vi "1726 Drive With PID.vi"(0 "RobotDriveDevRef in":T2, 1 "Tuning Parametres":T1 {"Acceleration Distance" min=0.0; "Minimum Speed" min=0.0 max=1.0; "Max Speed" min=0.0 max=1.0}, 2 "Target Distance":dbl, 3 "Timeout (ms)":u32) -> (7 "RobotDriveDevRef out":T2, 9 "Is Finished?":bool, 10 "Is Timedout?":bool)   [LabVIEW 2017]
uses:
  <vilib>/Rock Robotics/WPI/RobotDrive/WPI_RobotDriveDevRef.ctl
  <vilib>/Rock Robotics/WPI/MotorControl/WPI_MotorControlDeviceRef.ctl
  <vilib>/Rock Robotics/WPI/MotorControl/WPI_MotorControlType.ctl
  <vilib>/Rock Robotics/SystemInterfaces/DIO/FPGA_DIOPWMChannel.ctl
  <vilib>/Rock Robotics/WPI/PWM/WPI_PWMDeadband.ctl
  <vilib>/Rock Robotics/SystemInterfaces/DIO/FPGA_DIOChannel.ctl
  Team Code/Robot Global Data.vi
  <vilib>/addons/control/pid/pid.llb/PID (DBL).vi
  <vilib>/Rock Robotics/WPI/RobotDrive/WPI_RobotDriveArcadeDrive_Standard(NoSaturation).vi
  <vilib>/addons/control/pid/NI_PID_pid.lvlib
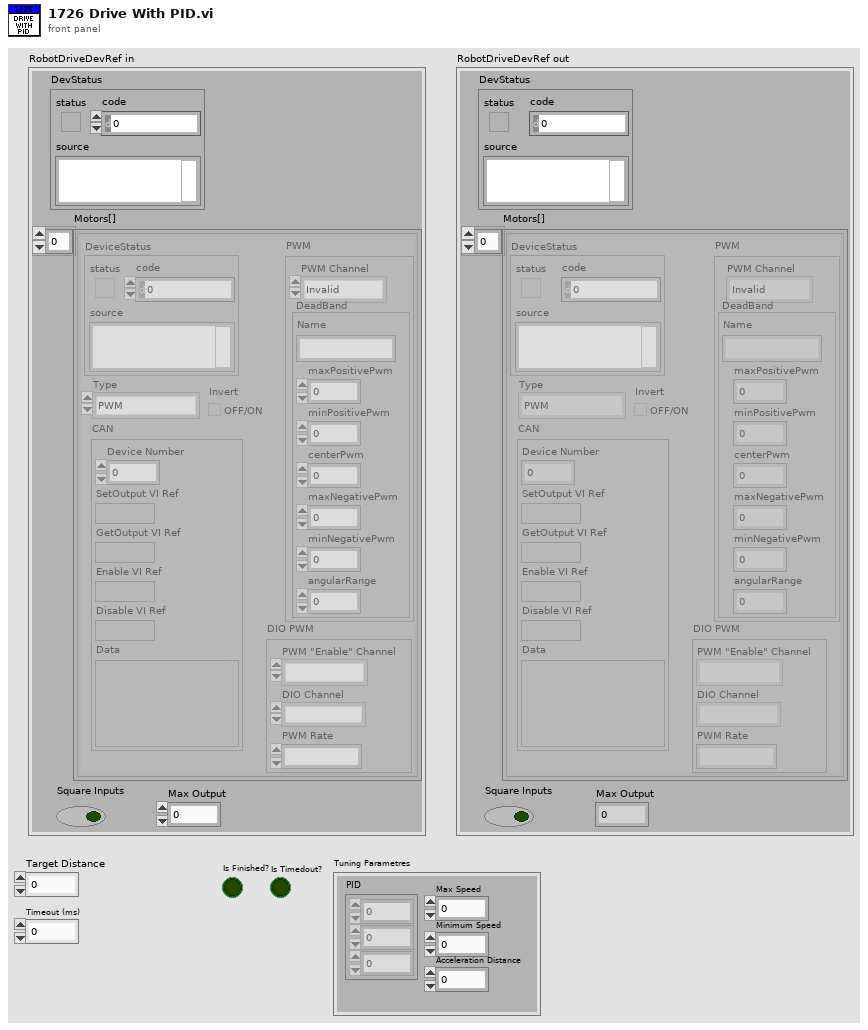
[diagram p1: front panel]
types:
  T1 = cluster{"PID":dbl[], "Max Speed":dbl, "Minimum Speed":dbl, "Acceleration Distance":dbl}
  T2 = typedef "WPI_RobotDriveDevRef.ctl" = cluster{"DevStatus":errorcluster, "Motors[]":T3[], "Square Inputs":bool, "Max Output":dbl}
  T3 = typedef "WPI_MotorControlDeviceRef.ctl" = cluster{"DeviceStatus":errorcluster, "Type":T4, "PWM":cluster{"PWM Channel":T5, "DeadBand":T6}, "CAN":cluster{"Device Number":u8, "SetOutput VI Ref":variant, "GetOutput VI Ref":variant, "Enable VI Ref":variant, "Disable VI Ref":variant, "Data":variant}, "Invert":bool, "DIO PWM":cluster{"PWM \"Enable\" Channel":T5, "DIOChannel":T7, "PWM Rate":dbl}}
  T4 = typedef "WPI_MotorControlType.ctl" = enum16{"PWM", "CAN", "DIO PWM"}
  T5 = typedef "FPGA_DIOPWMChannel.ctl" = enum8{"PWM 0", "PWM 1", "PWM 2", "PWM 3", "PWM 4", "PWM 5", "PWM 6", "PWM 7", "PWM 8", "PWM 9", "PWM MXP 0", "PWM MXP 1", "PWM MXP 2", "PWM MXP 3", "PWM MXP 4", "PWM MXP 5", "PWM MXP 6", "PWM MXP 7", "PWM MXP 8", "PWM MXP 9", "Invalid"}
  T6 = typedef "WPI_PWMDeadband.ctl" = cluster{"Name":string, "maxPositivePwm":i32, "minPositivePwm":i32, "centerPwm":i32, "maxNegativePwm":i32, "minNegativePwm":i32, "angularRange":u16}
  T7 = typedef "FPGA_DIOChannel.ctl" = enum8{"DIO 0", "DIO 1", "DIO 2", "DIO 3", "DIO 4", "DIO 5", "DIO 6", "DIO 7", "DIO 8", "DIO 9", "DIO MXP 0", "DIO MXP 1", "DIO MXP 2", "DIO MXP 3", "DIO MXP 4", "DIO MXP 5", "DIO MXP 6", "DIO MXP 7", "DIO MXP 8", "DIO MXP 9", "DIO MXP 10", "DIO MXP 11", "DIO MXP 12", "DIO MXP 13", "DIO MXP 14", "DIO MXP 15", "SPI Port CS1", "SPI Port CS2", "SPI Port CS3", "SPI Port MISO", "SPI Port MOSI", "Invalid"}
  T8 = cluster{"PID[0]":dbl, "PID[1]":dbl, "PID[2]":dbl}
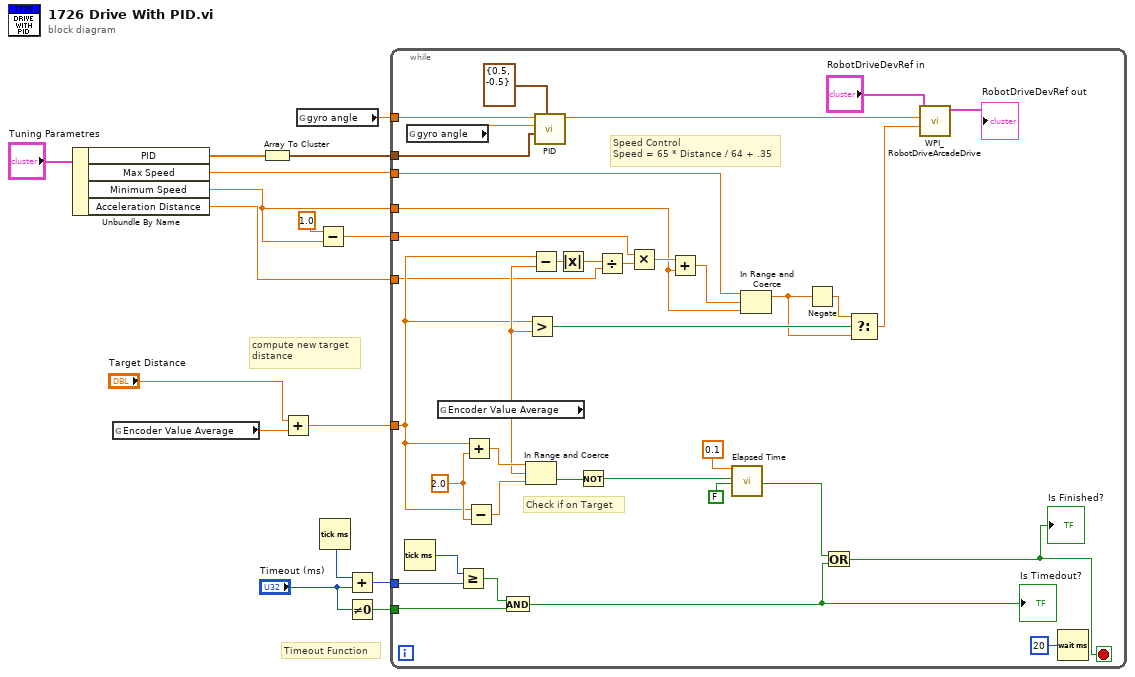
[diagram p0: block diagram]
diagram:
  # "Timeout Function"
  # "compute new target\ndistance"
  n1 = Unbundle By Name("Tuning Parametres") -> ("PID"=w6:dbl[], "Max Speed"=w5:dbl, "Minimum Speed"=w2:dbl, "Acceleration Distance"=w1:dbl)
  n2 = global read "Robot Global Data.vi" "Encoder Value Average"() -> (w14:dbl)
  n3 = Array To Cluster(array=w6) -> (cluster=w7:T8)
  n4 = Add(x="Target Distance", y=w14) -> (x+y=w13:dbl)
  n5 = global read "Robot Global Data.vi" "gyro angle"() -> (w16:dbl)
  n6 = Subtract(x=1.0, y=w2) -> (x-y=w3:dbl)
  n7 = Tick Count (ms)() -> (millisecond timer value=w12:u32)
  n8 = Add(x=w12, y="Timeout (ms)") -> (x+y=w11:u32)
  n9 = Not Equal To 0?(x="Timeout (ms)") -> (x != 0?=w9:bool)
  n10 = while {
    tunnel: w7 -> [w49]
    tunnel: w16 -> [w47]
    tunnel: w13 -> [w33]
    tunnel: w11 -> [w26]
    tunnel: w9 -> [w21]
    tunnel: w5 -> [w20]
    tunnel: w3 -> [w19]
    tunnel: w2 -> [w18]
    tunnel: w1 -> [w17]
    stop <- w24 stop-if-true
    w46 = 2.0 ("y")
    # "Check if on Target"
    # "Speed Control\nSpeed = 65 * Distance / 64 + .35"
    n11 = Tick Count (ms)() -> (millisecond timer value=w27:u32)
    n12 = global read "Robot Global Data.vi" "gyro angle"() -> (w48:dbl)
    n13 = global read "Robot Global Data.vi" "Encoder Value Average"() -> (w34:dbl)
    n14 = Greater Or Equal?(x=w27, y=w26) -> (x >= y?=w23:bool)
    n15 = Add(x=w33, y=w46) -> (x+y=w45:dbl)
    n16 = Subtract(x=w33, y=w46) -> (x-y=w44:dbl)
    n17 = And(x=w23, y=w21) -> (x .and. y?=w22:bool)
    "Is Timedout?" <- w22
    n18 = In Range and Coerce(upper limit=w45, x=w34, lower limit=w44) -> (In Range?=w41:bool)  [unwired: 1 out]
    n19 = Greater?(x=w33, y=w34) -> (0:w38:bool)
    n20 = Subtract(x=w33, y=w34) -> (x-y=w35:dbl)
    n21 = call-poly <vilib>:"PID.vi"("output range"=cluster{"output high":dbl, "output low":dbl} {"output high"=0.5, "output low"=-0.5}, "PID gains"=w49, "process variable"=w48, "setpoint"=w47) -> ("output"=w53:dbl)  [unwired: 6 in, 1 out]
    n22 = Absolute Value(x=w35) -> (abs(x)=w32:dbl)
    n23 = Not(x=w41) -> (.not. x?=w42:bool)
    n24 = Divide(x=w32, y=w17) -> (x/y=w36:dbl)
    n25 = Multiply(x=w19, y=w36) -> (x*y=w28:dbl)
    n26 = Add(x=w28, y=w18) -> (x+y=w31:dbl)
    n27 = call "Elapsed Time"("Time Target (s)"=0.1, "Reset"=w42, "Auto Reset"=FALSE) -> ("Time has Elapsed"=w25:bool)  [unwired: 9 in, 7 out]
    n28 = In Range and Coerce(upper limit=w20, x=w31, lower limit=w18) -> (coerced(x)=w29:dbl)  [unwired: 1 out]
    n29 = Negate(x=w29) -> (-x=w30:dbl)
    n30 = Or(x=w25, y=w22) -> (x .or. y?=w24:bool)
    "Is Finished?" <- w24
    n31 = Select(t=w30, s=w38, f=w29) -> (s? t:f=w37:dbl)
    n32 = call-poly <vilib>:"WPI_RobotDriveArcadeDrive.vi"("Y axis value"=w37, "X axis value"=w53, "RobotDriveDevRef"="RobotDriveDevRef in") -> ("RobotDriveDevRef"=→"RobotDriveDevRef out":T2)  [unwired: 1 in, 7 out]
    n33 = Wait (ms)(milliseconds to wait=u32 20) -> ()  [unwired: 1 out]
  }
